vi "Write CCD configuration.vi"(8 "error in (no error)":errorcluster, 10 "Camera Setup":T1={"Image Name"="Image", "# Images"=0, "Exposure Time"=0.0, "Pre-amp gain"=0, "Readout Rate"=0, "EM Mode"=0, "EM Gain"=2, "Vertical Binning"=1, "Horizontal Binning"=1, "Initial Line"=1, "Initial Cloumn"=1, "Final Line"=1024, "Final Column"=1024, "Kinetic Serie Length"=0, "Image path"="", "Shutter Mode"=2} {"Shutter Mode" items=["Auto", "Open", "Closed"]; "EM Mode" items=["Electron Multiplying", "Conventional"]; "Readout Rate" items=["1 MHz", "10 MHz", "20 MHz", "30 MHz"]; "Pre-amp gain" items=["Gain 1", "Gain 2"]}, 11 "CCD in":refnum<class "CCD.lvclass">) -> (0 "error out":errorcluster, 3 "CCD out":refnum<class "CCD.lvclass">)   [LabVIEW 2018, in "CCD.lvclass"]
uses:
  CCD.lvclass
  <userlib>/atmcd32d.llb/AcquisitionMode_mode typedef.ctl
  <userlib>/atmcd32d.llb/TriggerMode_mode typedef.ctl
  <userlib>/atmcd32d.llb/Shutter_type typedef.ctl
  <userlib>/atmcd32d.llb/ReadMode_mode typedef.ctl
  CCD.lvclass/CCD.ctl
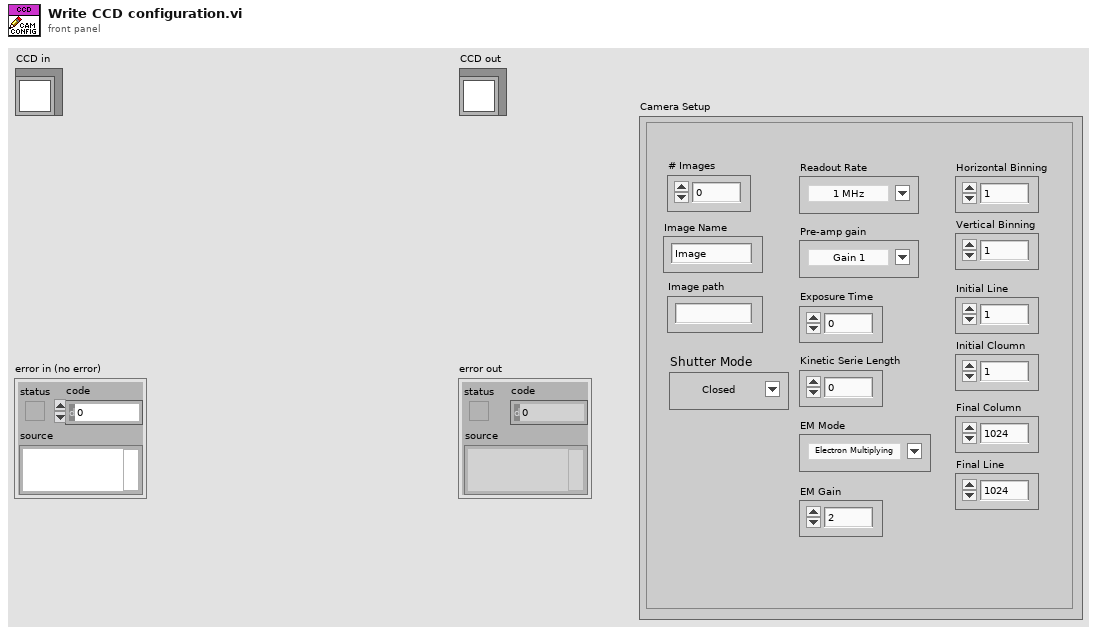
[diagram p1: front panel]
types:
  T1 = cluster{"Image Name":string, "# Images":u32, "Exposure Time":dbl, "Pre-amp gain":u8, "Readout Rate":u8, "EM Mode":u8, "EM Gain":u32, "Vertical Binning":u16, "Horizontal Binning":u16, "Initial Line":u16, "Initial Cloumn":u16, "Final Line":u16, "Final Column":u16, "Kinetic Serie Length":u32, "Image path":string, "Shutter Mode":u16}
  T2 = typedef "ReadMode_mode typedef.ctl" = enum16{"Full Vertical Binning", "Multi-Track", "Random-Track", "Single-Track", "Image"}
  T3 = typedef "Shutter_type typedef.ctl" = enum16{"TTL Low", "TTL High"}
  T4 = typedef "TriggerMode_mode typedef.ctl" = enum16{"Internal", "External", "N/A (2)", "N/A (3)", "N/A (4)", "N/A (5)", "External Start", "External Exposure (Bulb)", "N/A (8)", "External FVB EM", "Software", "N/A (11)", "External Charge Shifting"}
  T5 = typedef "AcquisitionMode_mode typedef.ctl" = enum16{"Reserved (0)", "Single Scan", "Accumulate", "Kinetics", "Fast Kinetics", "Run Till Abort", "Reserved (6)", "Reserved (7)", "Reserved (8)", "Time Delayed Integration"}
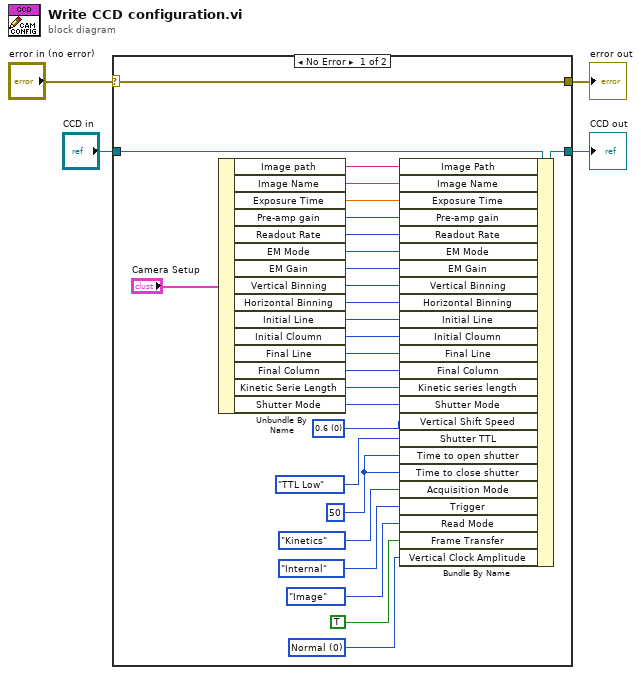
[diagram p0: block diagram]
diagram:
  n1 = case shown="No Error" "error in (no error)" {
    selector: "error in (no error)" -> [w31 w33]
    tunnel: [w31 w33] -> w3
    tunnel: [w7 w32] -> w1
    tunnel: "CCD in" -> [w16 w32]
    frame No Error {
      w13 = 50
      w8 = u8 0 items=["Normal", "+1", "+2", "+3", "+4"] ("Vertical Clock Amplitude")
      w15 = u8 0 items=["0.6", "1.13", "2.2", "4.33"] ("Vertical Shift Speed")
      n2 = Unbundle By Name("Camera Setup") -> ("Image path"=w6:string, "Image Name"=w29:string, "Exposure Time"=w28:dbl, "Pre-amp gain"=w27:u8, "Readout Rate"=w26:u8, "EM Mode"=w25:u8, "EM Gain"=w24:u32, "Vertical Binning"=w23:u16, "Horizontal Binning"=w22:u16, "Initial Line"=w21:u16, "Initial Cloumn"=w20:u16, "Final Line"=w19:u16, "Final Column"=w18:u16, "Kinetic Serie Length"=w17:u32, "Shutter Mode"=w5:u16)
      n3 = Bundle By Name(cluster=w16, "Image Path"=w6, "Image Name"=w29, "Exposure Time"=w28, "Pre-amp gain"=w27, "Readout Rate"=w26, "EM Mode"=w25, "EM Gain"=w24, "Vertical Binning"=w23, "Horizontal Binning"=w22, "Initial Line"=w21, "Initial Cloumn"=w20, "Final Line"=w19, "Final Column"=w18, "Kinetic series length"=w17, "Shutter Mode"=w5, "Vertical Shift Speed"=w15, "Shutter TTL"=Shutter_type_typedef."TTL Low" ("type"), "Time to open shutter"=w13, "Time to close shutter"=w13, "Acquisition Mode"=AcquisitionMode_mode_typedef."Kinetics" ("mode"), "Trigger"=TriggerMode_mode_typedef."Internal" ("mode"), "Read Mode"=ReadMode_mode_typedef."Image" ("mode"), "Frame Transfer"=TRUE, "Vertical Clock Amplitude"=w8) -> (w7:refnum<class "CCD.lvclass">)
    }
    frame Error {
    }
  }
  "error out" <- w3
  "CCD out" <- w1
